vi "插入温度记录.vi"   [LabVIEW 2022 SP3]
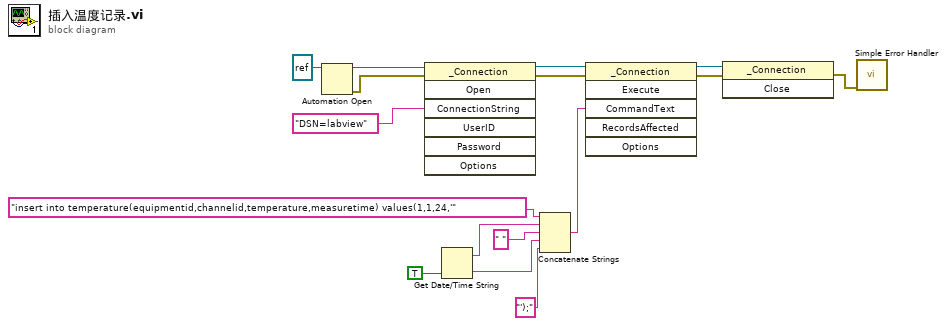
[diagram p0: block diagram]
diagram:
  n1 = Automation Open(Automation Refnum=refnum<k7> refnum ("ADODB._Connection")) -> (Automation Refnum=w15:refnum<k7>, error out=w14:errorcluster)  [unwired: 3 in]
  n2 = invoke class="_Connection" method="Open"(reference=w15, error in=w14, "ConnectionString"="DSN=labview") -> (reference out=w12:refnum<k7>, error out=w11:errorcluster)  [unwired: 4 in, 5 out]
  n3 = Get Date/Time String(want seconds? (F)=TRUE) -> (date string=w8:string, time string=w6:string)  [unwired: 2 in]
  n4 = Concatenate Strings("insert into temperature(equipmentid,channelid,temperature,measuretime) values(1,1,24,'" ("CommandText"), w8, " " ("string"), w6, "');" ("string")) -> (w4:string)
  n5 = invoke class="_Connection" method="Execute"(reference=w12, error in=w11, "CommandText"=w4) -> (reference out=w3:refnum<k7>, error out=w2:errorcluster)  [unwired: 3 in, 4 out]
  n6 = invoke class="_Connection" method="Close"(reference=w3, error in=w2) -> (error out=w1:errorcluster)  [unwired: 1 in, 2 out]
  n7 = call <vilib>:"Simple Error Handler.vi"("error in (no error)"=w1) -> ()  [unwired: 4 in, 5 out]
